vi "Set Sample Rate.vi"(8 "error in (no error)":errorcluster, 10 "Sample Rate (100 Hz)":u16=100 min=1 max=1000 step=1, 11 "VISA resource name":refnum<visa-resource-name>) -> (0 "error out":errorcluster, 3 "VISA resource name out":refnum<visa-resource-name>)   [LabVIEW 2012, in "MicroStrain 3DM-GXx.lvlib"]
doc: "Set the rate at which the device returns data. Valid sample rates are between 1 and 1000Hz. The VI also configures the appropriate baud rate to ensure the input sample rate."
uses:
  <instrlib>/MicroStrain 3DM-GXx/MicroStrain 3DM-GXx.lvlib
  <vilib>/Instr/_visa.llb/VISA Configure Serial Port (Instr).vi
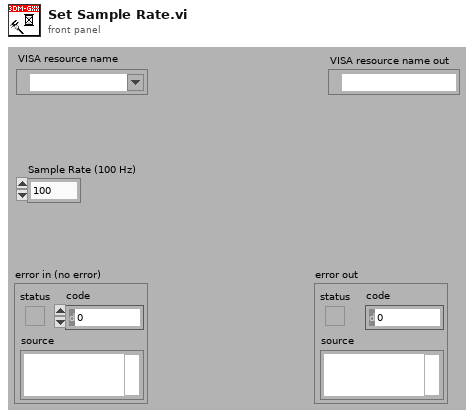
[diagram p1: front panel]
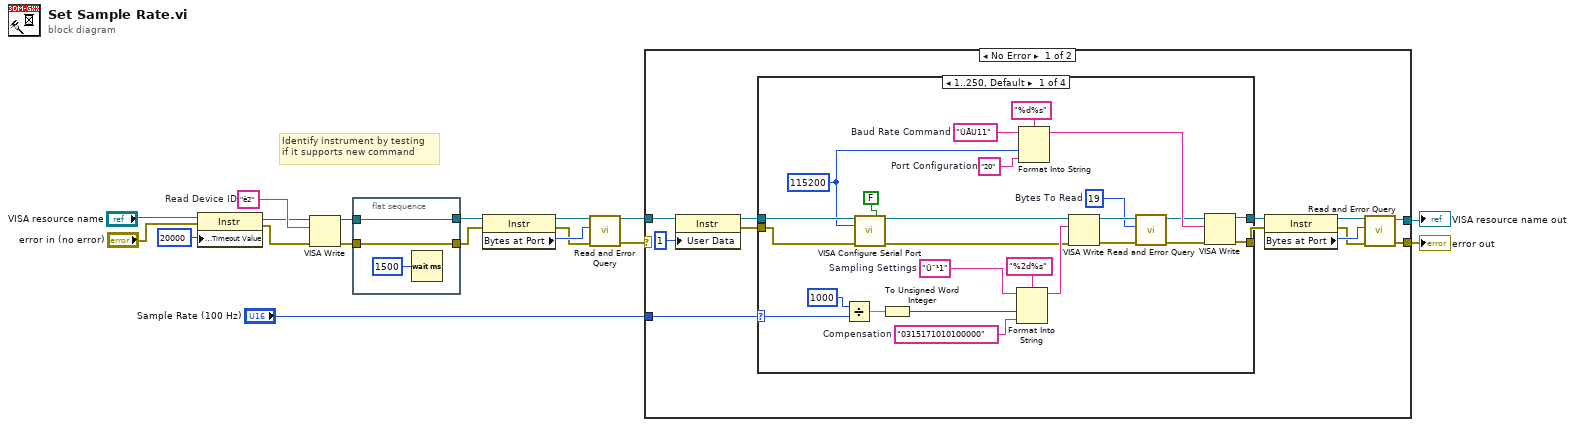
[diagram p0: block diagram]
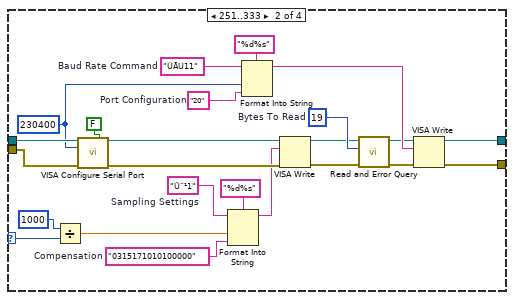
[diagram p2: hidden frame]
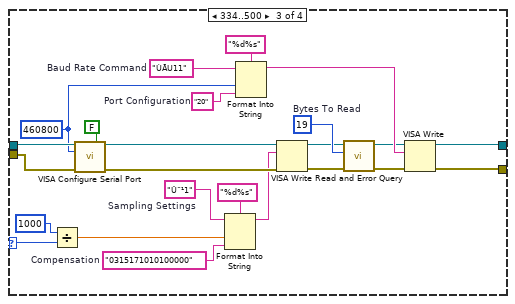
[diagram p3: hidden frame]
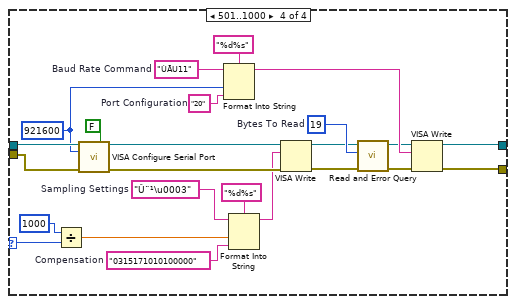
[diagram p4: hidden frame]
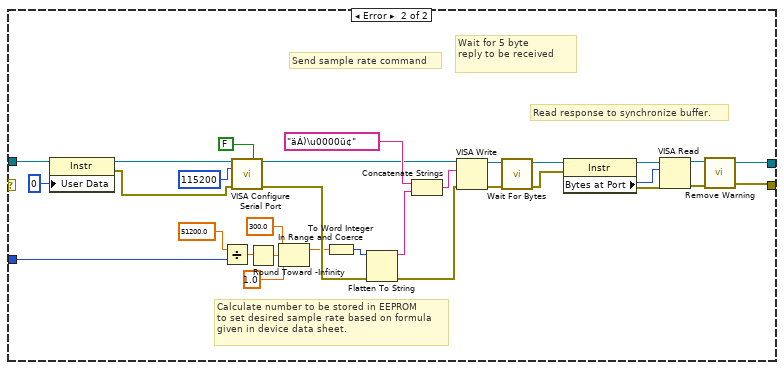
[diagram p5: hidden frame]
diagram:
  w17 = "ê2"  # Read Device ID
  # "Identify instrument by testing\nif it supports new command"
  n1 = property class="Instr"(reference="VISA resource name", error in="error in (no error)", "General Settings:Timeout Value"=u32 20000) -> (reference out=w9:refnum<visa-resource-name>, error out=w8:errorcluster)
  n2 = VISA Write(VISA resource name=w9, write buffer=w17, error in (no error)=w8) -> (VISA resource name out=w7:refnum<visa-resource-name>, error out=w6:errorcluster)  [unwired: 1 out]
  n3 = flat-sequence {
    tunnel: w7 -> [w20]
    tunnel: w6 -> [w19]
    tunnel: [w20] -> w5
    tunnel: [w19] -> w4
    frame #0 {
      n4 = Wait (ms)(milliseconds to wait=u32 1500) -> ()  [unwired: 1 out]
    }
  }
  n5 = property class="Instr"(reference=w5, error in=w4) -> (reference out=w3:refnum<visa-resource-name>, error out=w1:errorcluster, "Bytes at Port"=w2:u32)
  n6 = call <instrlib>:"Read and Error Query.vi"("error in (no error)"=w1, "Bytes To Read (0)"=w2, "VISA resource name"=w3) -> ("error out"=w13:errorcluster, "VISA resource name out"=w14:refnum<visa-resource-name>)  [unwired: 7 in]
  n7 = case shown="No Error" w13 {
    tunnel: "Sample Rate (100 Hz)" -> [w33 w153]
    tunnel: w14 -> [w24 w139]
    tunnel: [w27 w145] -> w15
    tunnel: [w26 w144] -> w16
    frame No Error {
      n8 = property class="Instr"(reference=w24, "User Data"=u32 1 ("General Settings:User Data")) -> (reference out=w23:refnum<visa-resource-name>, error out=w22:errorcluster)  [unwired: 1 in]
      n9 = case shown="1..250, Default" w33 {
        selector: w33 -> [w57 w72 w96 w120]
        tunnel: w23 -> [w39 w73 w97 w121]
        tunnel: [w48 w66 w90 w114] -> w32
        tunnel: [w47 w65 w89 w113] -> w31
        tunnel: w22 -> [w38 w59 w83 w107]
        frame 1..250, Default {
          w34 = u32 115200 ("baud rate (9600)")
          w42 = u32 19  # Bytes To Read
          w51 = "20"  # Port Configuration
          w52 = "ÙÃU11"  # Baud Rate Command
          w55 = "0315171010100000"  # Compensation
          w56 = "Û¨¹1"  # Sampling Settings
          n10 = Divide(x=1000, y=w57) -> (x/y=w46:dbl)
          n11 = call-poly "VISA Configure Serial Port"("VISA resource name"=w39, "Enable Termination\nChar (T)"=FALSE ("Enable Termination\nChar (T)"), "baud rate (9600)"=w34, "error in (no error)"=w38) -> ("VISA resource name out"=w36:refnum<visa-resource-name>, "error out"=w35:errorcluster)  [unwired: 10 in]
          n12 = To Unsigned Word Integer(number=w46) -> (unsigned 16bit integer=w45:u16)
          n13 = Format Into String(format string="%2d%s", initial string=w56, w45, w55) -> (resulting string=w53:string)  [unwired: 1 in, 1 out]
          n14 = Format Into String(format string="%d%s", initial string=w52, w34, w51) -> (resulting string=w49:string)  [unwired: 1 in, 1 out]
          n15 = VISA Write(VISA resource name=w36, write buffer=w53, error in (no error)=w35) -> (VISA resource name out=w44:refnum<visa-resource-name>, error out=w43:errorcluster)  [unwired: 1 out]
          n16 = call <instrlib>:"Read and Error Query.vi"("error in (no error)"=w43, "Bytes To Read (0)"=w42, "VISA resource name"=w44) -> ("error out"=w40:errorcluster, "VISA resource name out"=w41:refnum<visa-resource-name>)  [unwired: 7 in]
          n17 = VISA Write(VISA resource name=w41, write buffer=w49, error in (no error)=w40) -> (VISA resource name out=w48:refnum<visa-resource-name>, error out=w47:errorcluster)  [unwired: 1 out]
        }
        frame 251..333 {
          w64 = u32 19  # Bytes To Read
          w70 = "20"  # Port Configuration
          w71 = "ÙÃU11"  # Baud Rate Command
          w76 = "0315171010100000"  # Compensation
          w77 = "Û¨¹1"  # Sampling Settings
          w69 = u32 230400 ("baud rate (9600)")
          n18 = Divide(x=1000, y=w72) -> (x/y=w78:dbl)
          n19 = call-poly "VISA Configure Serial Port"("VISA resource name"=w73, "Enable Termination\nChar (T)"=FALSE ("Enable Termination\nChar (T)"), "baud rate (9600)"=w69, "error in (no error)"=w59) -> ("VISA resource name out"=w80:refnum<visa-resource-name>, "error out"=w79:errorcluster)  [unwired: 10 in]
          n20 = Format Into String(format string="%d%s", initial string=w77, w78, w76) -> (resulting string=w74:string)  [unwired: 1 in, 1 out]
          n21 = Format Into String(format string="%d%s", initial string=w71, w69, w70) -> (resulting string=w67:string)  [unwired: 1 in, 1 out]
          n22 = VISA Write(VISA resource name=w80, write buffer=w74, error in (no error)=w79) -> (VISA resource name out=w63:refnum<visa-resource-name>, error out=w62:errorcluster)  [unwired: 1 out]
          n23 = call <instrlib>:"Read and Error Query.vi"("error in (no error)"=w62, "Bytes To Read (0)"=w64, "VISA resource name"=w63) -> ("error out"=w60:errorcluster, "VISA resource name out"=w61:refnum<visa-resource-name>)  [unwired: 7 in]
          n24 = VISA Write(VISA resource name=w61, write buffer=w67, error in (no error)=w60) -> (VISA resource name out=w66:refnum<visa-resource-name>, error out=w65:errorcluster)  [unwired: 1 out]
        }
        frame 334..500 {
          w88 = u32 19  # Bytes To Read
          w94 = "20"  # Port Configuration
          w95 = "ÙÃU11"  # Baud Rate Command
          w100 = "0315171010100000"  # Compensation
          w101 = "Û¨¹1"  # Sampling Settings
          w93 = u32 460800 ("baud rate (9600)")
          n25 = Divide(x=1000, y=w96) -> (x/y=w102:dbl)
          n26 = call-poly "VISA Configure Serial Port"("VISA resource name"=w97, "Enable Termination\nChar (T)"=FALSE ("Enable Termination\nChar (T)"), "baud rate (9600)"=w93, "error in (no error)"=w83) -> ("VISA resource name out"=w104:refnum<visa-resource-name>, "error out"=w103:errorcluster)  [unwired: 10 in]
          n27 = Format Into String(format string="%d%s", initial string=w101, w102, w100) -> (resulting string=w98:string)  [unwired: 1 in, 1 out]
          n28 = Format Into String(format string="%d%s", initial string=w95, w93, w94) -> (resulting string=w91:string)  [unwired: 1 in, 1 out]
          n29 = VISA Write(VISA resource name=w104, write buffer=w98, error in (no error)=w103) -> (VISA resource name out=w87:refnum<visa-resource-name>, error out=w86:errorcluster)  [unwired: 1 out]
          n30 = call <instrlib>:"Read and Error Query.vi"("error in (no error)"=w86, "Bytes To Read (0)"=w88, "VISA resource name"=w87) -> ("error out"=w84:errorcluster, "VISA resource name out"=w85:refnum<visa-resource-name>)  [unwired: 7 in]
          n31 = VISA Write(VISA resource name=w85, write buffer=w91, error in (no error)=w84) -> (VISA resource name out=w90:refnum<visa-resource-name>, error out=w89:errorcluster)  [unwired: 1 out]
        }
        frame 501..1000 {
          w112 = u32 19  # Bytes To Read
          w118 = "20"  # Port Configuration
          w119 = "ÙÃU11"  # Baud Rate Command
          w124 = "0315171010100000"  # Compensation
          w125 = "Û¨¹\u0003"  # Sampling Settings
          w117 = u32 921600 ("baud rate (9600)")
          n32 = Divide(x=1000, y=w120) -> (x/y=w126:dbl)
          n33 = call-poly "VISA Configure Serial Port"("VISA resource name"=w121, "Enable Termination\nChar (T)"=FALSE ("Enable Termination\nChar (T)"), "baud rate (9600)"=w117, "error in (no error)"=w107) -> ("VISA resource name out"=w128:refnum<visa-resource-name>, "error out"=w127:errorcluster)  [unwired: 10 in]
          n34 = Format Into String(format string="%d%s", initial string=w119, w117, w118) -> (resulting string=w115:string)  [unwired: 1 in, 1 out]
          n35 = Format Into String(format string="%d%s", initial string=w125, w126, w124) -> (resulting string=w122:string)  [unwired: 1 in, 1 out]
          n36 = VISA Write(VISA resource name=w128, write buffer=w122, error in (no error)=w127) -> (VISA resource name out=w111:refnum<visa-resource-name>, error out=w110:errorcluster)  [unwired: 1 out]
          n37 = call <instrlib>:"Read and Error Query.vi"("error in (no error)"=w110, "Bytes To Read (0)"=w112, "VISA resource name"=w111) -> ("error out"=w108:errorcluster, "VISA resource name out"=w109:refnum<visa-resource-name>)  [unwired: 7 in]
          n38 = VISA Write(VISA resource name=w109, write buffer=w115, error in (no error)=w108) -> (VISA resource name out=w114:refnum<visa-resource-name>, error out=w113:errorcluster)  [unwired: 1 out]
        }
      }
      n39 = property class="Instr"(reference=w32, error in=w31) -> (reference out=w29:refnum<visa-resource-name>, error out=w28:errorcluster, "Bytes at Port"=w30:u32)
      n40 = call <instrlib>:"Read and Error Query.vi"("error in (no error)"=w28, "Bytes To Read (0)"=w30, "VISA resource name"=w29) -> ("error out"=w26:errorcluster, "VISA resource name out"=w27:refnum<visa-resource-name>)  [unwired: 7 in]
    }
    frame Error {
      # "Wait for 5 byte\nreply to be received"
      # "Read response to synchronize buffer."
      # "Send sample rate command"
      # "Calculate number to be stored in EEPROM\nto set desired sample rate based on formula\ngiven in device data sheet."
      n41 = property class="Instr"(reference=w139, "User Data"=u32 0 ("General Settings:User Data")) -> (reference out=w138:refnum<visa-resource-name>, error out=w137:errorcluster)  [unwired: 1 in]
      n42 = Divide(x=51200.0, y=w153) -> (x/y=w161:dbl)
      n43 = call-poly "VISA Configure Serial Port"("VISA resource name"=w138, "Enable Termination\nChar (T)"=FALSE ("Enable Termination\nChar (T)"), "baud rate (9600)"=u32 115200, "error in (no error)"=w137) -> ("VISA resource name out"=w147:refnum<visa-resource-name>, "error out"=w146:errorcluster)  [unwired: 10 in]
      n44 = Round Toward -Infinity(1:w161) -> (0:w141:dbl)
      n45 = In Range and Coerce(upper limit=300.0, x=w141, lower limit=1.0) -> (coerced(x)=w140:dbl)  [unwired: 1 out]
      n46 = To Word Integer(number=w140) -> (16bit integer=w159:i16)
      n47 = Flatten To String(anything=w159, error in (no error)=w146) -> (data string=w157:string, error out=w152:errorcluster)  [unwired: 2 in, 1 out]
      n48 = Concatenate Strings("äÁ)\u0000ü¢" ("write buffer"), w157) -> (w154:string)
      n49 = VISA Write(VISA resource name=w147, write buffer=w154, error in (no error)=w152) -> (VISA resource name out=w156:refnum<visa-resource-name>, error out=w155:errorcluster)  [unwired: 1 out]
      n50 = call <instrlib>:"Wait For Bytes.vi"("error in (no error)"=w155, "VISA resource name"=w156) -> ("error out"=w134:errorcluster, "VISA resource name out"=w135:refnum<visa-resource-name>)  [unwired: 8 in]
      n51 = property class="Instr"(reference=w135, error in=w134) -> (reference out=w133:refnum<visa-resource-name>, error out=w132:errorcluster, "Bytes at Port"=w131:u32)
      n52 = VISA Read(VISA resource name=w133, byte count=w131, error in (no error)=w132) -> (VISA resource name out=w151:refnum<visa-resource-name>, error out=w150:errorcluster)  [unwired: 2 out]
      n53 = call <instrlib>:"Remove Warning.vi"("error in (no error)"=w150, "VISA resource name"=w151) -> ("error out"=w144:errorcluster, "VISA resource name out"=w145:refnum<visa-resource-name>)  [unwired: 2 in]
    }
  }
  "VISA resource name out" <- w15
  "error out" <- w16
